vi "saveRowColor.vi"(8 "error in (no error)":errorcluster, 11 "reference in":refnum<class "Project Panels.lvclass">) -> (0 "error out":errorcluster, 3 "reference out":refnum<class "Project Panels.lvclass">)   [LabVIEW 2014, in "Project Panels.lvclass"]
uses:
  Project Panels.lvclass
  APP/excelFile_class/fileType.ctl
  SYS/File Controller_llb/File Controller.lvclass
  APP/excelFile_class/excelFile.lvclass
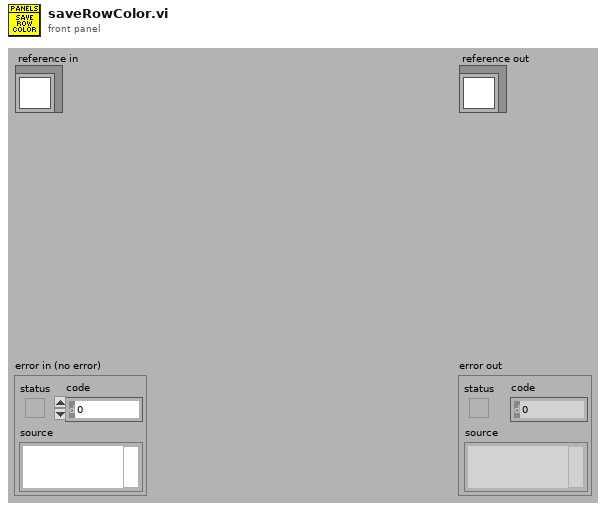
[diagram p1: front panel]
types:
  T1 = typedef "excelFile.lvclass/fileType.ctl" = enum16{"devices", "items", "partsTracking"}
  T2 = typedef "Project Panels.lvclass/ObjectAttributesRef.ctl" = refnum<data-value>
  T3 = typedef "Project Panels.lvclass/ObjectAttributes.ctl" = cluster{"MyAttribute":dbl, "device_controller_ref":refnum<class "Devices Controller.lvclass">, "file_controller_ref":refnum<class "File Controller.lvclass">, "item_controller_ref":refnum<class "Items Controller.lvclass">, "item_tables":cluster{"checkIN":string[][], "checkOUT":string[][], "storage":string[][]}, "quickbook_table":cluster{"notes":string[][]}, "notification_controller_ref":refnum<class "Notification Controller.lvclass">, "partstracking_controller_ref":refnum<class "PartsTracking Controller.lvclass">, "product_tables":cluster{"k4b2":string[][], "fitmate":string[][], "RMR":string[][], "CPET":string[][], "BP":string[][], "PP":string[][], "k5":string[][], "bb-pft":string[][]}, "rowsColour":u32[]}
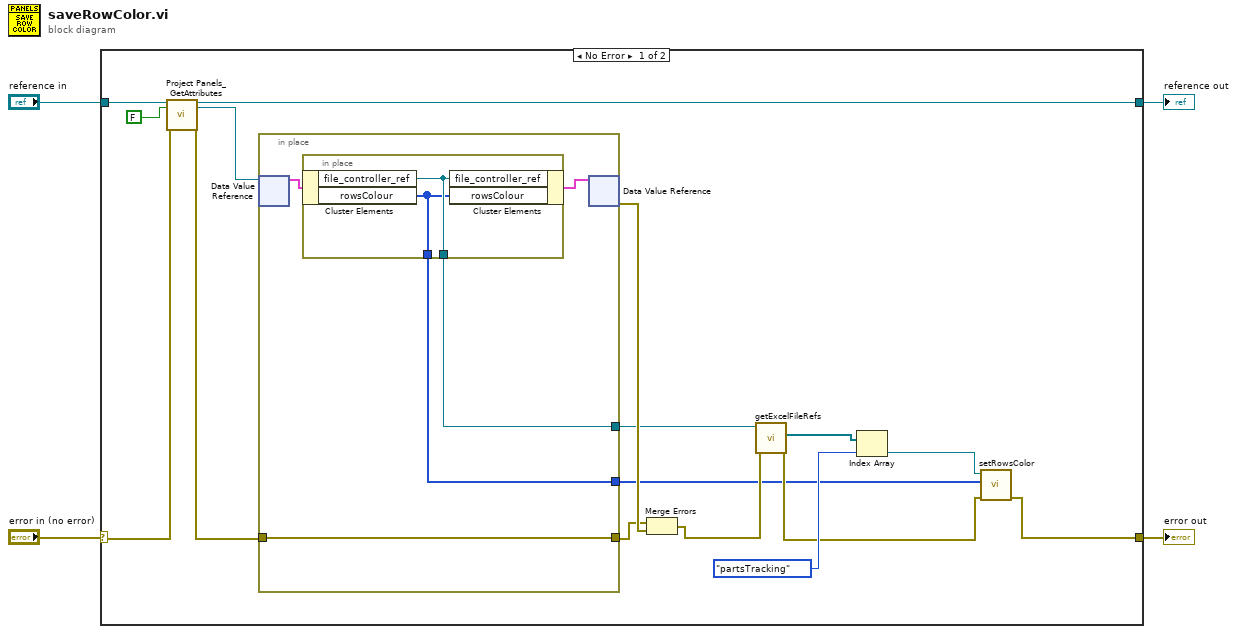
[diagram p0: block diagram]
diagram:
  n1 = case shown="No Error" "error in (no error)" {
    selector: "error in (no error)" -> [w16 w29]
    tunnel: [w7 w29] -> w3
    tunnel: [w14 w28] -> w1
    tunnel: "reference in" -> [w18 w28]
    frame No Error {
      n2 = call "Project Panels_GetAttributes.vi"("reference in"=w18, "return data? (T)"=FALSE, "error in (no error)"=w16) -> ("reference out"=w14:refnum<class "Project Panels.lvclass">, "attributes ref"=w13:T2, "error out"=w15:errorcluster)  [unwired: 13 in, 1 out]
      n3 = in-place {
        in-place-border: w15 -> [w23]
        in-place-border: [w23] -> w19
        in-place-border: [w22] -> w6
        in-place-border: [w21] -> w5
        n4 = in-place-dvr #1(w13) -> (w24:T3)  [unwired: 1 out]
        n5 = in-place {
          in-place-border: [w27] -> w22
          in-place-border: [w26] -> w21
          n6 = in-place-cluster #2(w24) -> ("file_controller_ref"=w27:refnum<class "File Controller.lvclass">, "rowsColour"=w26:u32[])
          n7 = in-place-cluster #2("file_controller_ref"=w27, "rowsColour"=w26) -> (w25:T3)
        }
        n8 = in-place-dvr #1(w25) -> (w20:errorcluster)  [unwired: 1 out]
      }
      n9 = Merge Errors(w19, w20) -> (w8:errorcluster)
      n10 = call "getExcelFileRefs.vi"("error in (no error)"=w8, "reference in"=w6) -> ("error out"=w10:errorcluster, "excelFile_refs"=w12:refnum<class "excelFile.lvclass">[])  [unwired: 7 in, 1 out]
      n11 = Index Array(array=w12, index=fileType."partsTracking" ("fileType")) -> (element=w9:refnum<class "excelFile.lvclass">)
      n12 = call "setRowsColor.vi"("error in (no error)"=w10, "rowsColor"=w5, "reference in"=w9) -> ("error out"=w7:errorcluster)  [unwired: 7 in, 1 out]
    }
    frame Error {
    }
  }
  "error out" <- w3
  "reference out" <- w1
